vi "Create Result Rows.vi"(10 "Values":refnum<class "Type.lvclass">[][](array[class]), 11 "Database in":refnum<class "Database Platform.lvclass">) -> (1 "Results":refnum<class "Result Row.lvclass">[](array[class]), 3 "Database out":refnum<class "Database Platform.lvclass">)   [LabVIEW 2020, in "Conditum.lvlib" / "Database Platform.lvclass"]
uses:
  Database Platform.lvclass
  Result Row/Result Row.lvclass
  Columns/Type/Type.lvclass
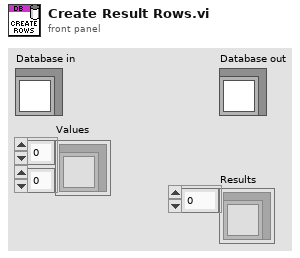
[diagram p1: front panel]
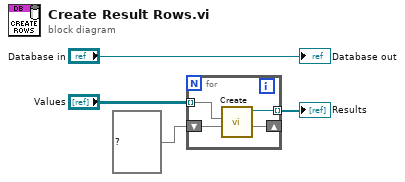
[diagram p0: block diagram]
diagram:
  n1 = for {
    tunnel: [w8] -> w3 mode=indexing
    tunnel: "Values" -> [w7] mode=indexing
    shift-right: [w6] -> _
    shift-left: map{string, i32} {} ("Name Map") -> [w5]
    n2 = call "Create.vi"("Name Map In"=w5, "Values"=w7) -> ("Name Map"=w6:map{string, i32}, "Result Row out"=w8:refnum<class "Result Row.lvclass">)  [unwired: 7 in, 1 out]
  }
  "Results" <- w3
  "Database out" <- "Database in"
